vi "RI plotter.vi"(0 "Resistance val":refnum<vi>, 1 "Resistance Indicator":refnum<vi>, 3 "Current Indicator":refnum<vi>, 5 "Current val":refnum<vi>, 9 "Detection Thr [%]":refnum<vi>, 11 "error in":errorcluster, 12 "R0":refnum<vi>, 13 "R2":refnum<vi>, 14 "Exit":refnum<vi>) -> (15 "error out":errorcluster)   [LabVIEW 2012, in "Signal Analysis.lvlib"]
uses:
  Signal Analysis.lvlib
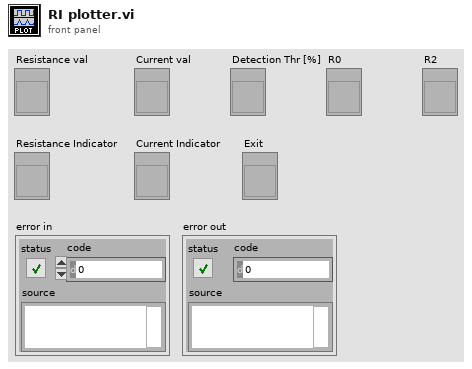
[diagram p1: front panel]
types:
  T1 = cluster{"Value":dbl, "Value 2":dbl, "Value 3":dbl}
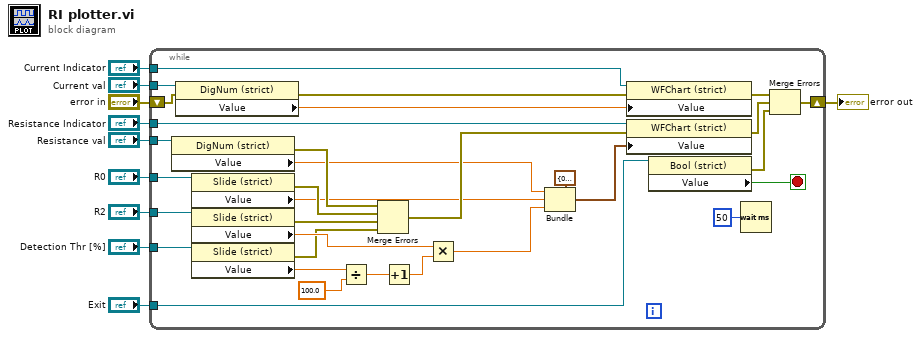
[diagram p0: block diagram]
diagram:
  n1 = while {
    tunnel: "Resistance val" -> [w42]
    tunnel: "Resistance Indicator" -> [w41]
    tunnel: "R0" -> [w40]
    tunnel: "Current val" -> [w38]
    tunnel: "Current Indicator" -> [w37]
    shift-right: [w33] -> w5
    shift-left: "error in" -> [w35]
    tunnel: "Exit" -> [w28]
    tunnel: "R2" -> [w19]
    tunnel: "Detection Thr [%]" -> [w18]
    stop <- w26 stop-if-true
    n2 = property class="DigNum (strict)"(reference=w42) -> (error out=w31:errorcluster, "Value"=w24:dbl)  [unwired: 1 in, 1 out]
    n3 = property class="DigNum (strict)"(reference=w38, error in=w35) -> (error out=w36:errorcluster, "Value"=w39:dbl)  [unwired: 1 out]
    n4 = property class="Slide (strict)"(reference=w40) -> (error out=w30:errorcluster, "Value"=w20:dbl)  [unwired: 1 in, 1 out]
    n5 = property class="Slide (strict)"(reference=w19) -> (error out=w15:errorcluster, "Value"=w17:dbl)  [unwired: 1 in, 1 out]
    n6 = property class="Slide (strict)"(reference=w18) -> (error out=w14:errorcluster, "Value"=w13:dbl)  [unwired: 1 in, 1 out]
    n7 = Divide(x=w13, y=100.0) -> (x/y=w21:dbl)
    n8 = Merge Errors(w31, w30, w15, w14) -> (w29:errorcluster)
    n9 = Increment(x=w21) -> (x+1=w12:dbl)
    n10 = Multiply(x=w17, y=w12) -> (x*y=w11:dbl)
    n11 = Bundle(cluster=T1 {"Value"=0.0, "Value 2"=0.0, "Value 3"=0.0}, "Value"=w24, "Value 2"=w20, "Value 3"=w11) -> (w22:T1)
    n12 = property class="WFChart (strict)"(reference=w37, error in=w36, "Value"=w39) -> (error out=w34:errorcluster)  [unwired: 1 out]
    n13 = property class="WFChart (strict)"(reference=w41, error in=w29, "Value"=w22) -> (error out=w32:errorcluster)  [unwired: 1 out]
    n14 = property class="Bool (strict)"(reference=w28) -> (error out=w27:errorcluster, "Value"=w26:bool)  [unwired: 1 in, 1 out]
    n15 = Wait (ms)(milliseconds to wait=u32 50) -> ()  [unwired: 1 out]
    n16 = Merge Errors(w34, w32, w27) -> (w33:errorcluster)
  }
  "error out" <- w5
